vi "公式波形.vi"() -> ()   [LabVIEW 2018]
uses:
  <vilib>/measure/NI_MAPro.lvlib
panel:
  in  "停止":bool
  out "波形图":waveform(dbl)(graph)
  in  "组合框":string(combo)
  in  "sampling info":cluster{"Fs":dbl, "#s":dbl}={"Fs"=1000.0, "#s"=1000.0} caption="采样信息" {"Fs" format="%.2p"}
  in  "reset signal":bool caption="重置信号"
  in  "amplitude":dbl=1.0 caption="幅值" format="%0.2p"
  in  "frequency":dbl=10.0 caption="频率" format="%0.2p"
  out "字符串":string="公式波形：用公式字符串指定要使用的时间函数"
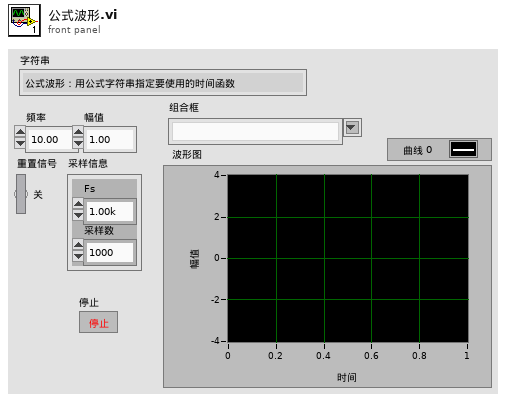
[diagram p1: front panel]
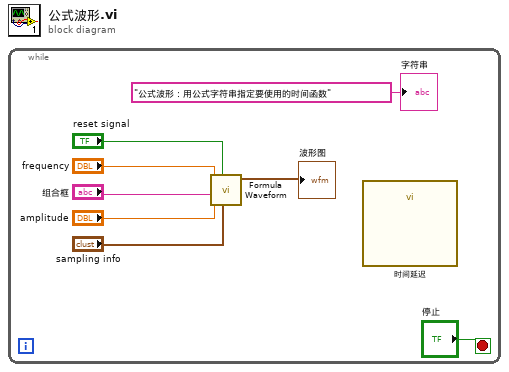
[diagram p0: block diagram]
diagram:
  n1 = while {
    stop <- "停止" stop-if-true
    n2 = call <vilib>:"Formula Waveform.vi"("sampling info"="sampling info", "reset signal"="reset signal", "formula"="组合框", "amplitude"="amplitude", "frequency"="frequency") -> ("signal out"=→"波形图":waveform(dbl))  [unwired: 5 in, 1 out]
    n3 = call "时间延迟"() -> ()  [unwired: 11 in, 1 out]
    "字符串" <- "公式波形：用公式字符串指定要使用的时间函数"
  }
